vi "Driver Controller.vi"   [LabVIEW 2018]
uses:
  <vilib>/Rock Robotics/WPI/Joystick/WPI_JoystickDeviceEnum.ctl
  Driver Controller Global.vi
types:
  T1 = typedef "WPI_JoystickDeviceEnum.ctl" = enum16{"USB 0", "USB 1", "USB 2", "USB 3", "USB 4", "USB 5"}
  T2 = typedef "WPI_JoystickDevRef.ctl" = cluster{"Device":T1}
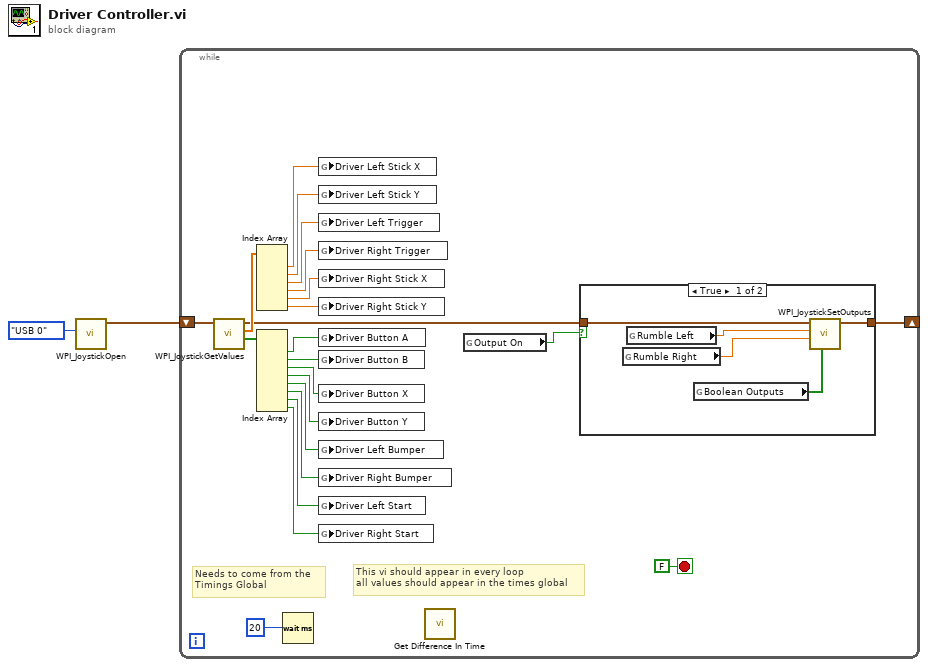
[diagram p0: block diagram]
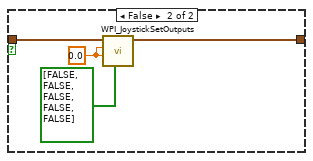
[diagram p2: hidden frame]
diagram:
  n1 = call <vilib>:"WPI_JoystickOpen.vi"("JoystickDevice"=WPI_JoystickDeviceEnum."USB 0") -> ("JoystickDevRef"=w1:T2)  [unwired: 10 in]
  n2 = while {
    shift-right: [w5] -> _
    shift-left: w1 -> [w24]
    stop <- FALSE stop-if-true
    # "This vi should appear in every loop\nall values should appear in the times global"
    # "Needs to come from the\nTimings Global"
    n3 = call <vilib>:"WPI_JoystickGetValues.vi"("JoystickDevRef"=w24) -> ("Buttons"=w16:bool[], "Axes"=w23:dbl[], "JoystickDevRef"=w4:T2)  [unwired: 6 in, 2 out]
    n4 = Index Array(array=w23) -> (element #1=w22:dbl, element #2=w21:dbl, element #3=w20:dbl, element #4=w19:dbl, element #5=w18:dbl, element #6=w17:dbl)  [unwired: 6 in]
    n5 = Index Array(array=w16) -> (element #1=w15:bool, element #2=w14:bool, element #3=w13:bool, element #4=w12:bool, element #5=w11:bool, element #6=w10:bool, element #7=w9:bool, element #8=w8:bool)  [unwired: 8 in]
    n6 = Wait (ms)(milliseconds to wait=20) -> ()  [unwired: 1 out]
    n7 = global write "Driver Controller Global.vi" "Driver Left Stick X"(w22) -> ()
    n8 = global write "Driver Controller Global.vi" "Driver Left Stick Y"(w21) -> ()
    n9 = global write "Driver Controller Global.vi" "Driver Left Trigger"(w20) -> ()
    n10 = global write "Driver Controller Global.vi" "Driver Right Trigger"(w19) -> ()
    n11 = global write "Driver Controller Global.vi" "Driver Right Stick X"(w18) -> ()
    n12 = global write "Driver Controller Global.vi" "Driver Right Stick Y"(w17) -> ()
    n13 = global write "Driver Controller Global.vi" "Driver Button A"(w15) -> ()
    n14 = global write "Driver Controller Global.vi" "Driver Button B"(w14) -> ()
    n15 = global write "Driver Controller Global.vi" "Driver Button X"(w13) -> ()
    n16 = global write "Driver Controller Global.vi" "Driver Button Y"(w12) -> ()
    n17 = global write "Driver Controller Global.vi" "Driver Left Bumper"(w11) -> ()
    n18 = global write "Driver Controller Global.vi" "Driver Right Bumper"(w10) -> ()
    n19 = global write "Driver Controller Global.vi" "Driver Left Start"(w9) -> ()
    n20 = global write "Driver Controller Global.vi" "Driver Right Start"(w8) -> ()
    n21 = call "Get Difference In Time.vi"() -> ()  [unwired: 10 in, 2 out]
    n22 = global read "Driver Controller Global.vi" "Output On"() -> (w3:bool)
    n23 = case shown="True" w3 {
      tunnel: [w29 w33] -> w5
      tunnel: w4 -> [w28 w32]
      frame True {
        n24 = global read "Driver Controller Global.vi" "Rumble Right"() -> (w26:dbl)
        n25 = global read "Driver Controller Global.vi" "Rumble Left"() -> (w27:dbl)
        n26 = global read "Driver Controller Global.vi" "Boolean Outputs"() -> (w25:bool[])
        n27 = call <vilib>:"WPI_JoystickSetOutputs.vi"("Outputs"=w25, "Right Rumble"=w26, "Left Rumble"=w27, "JoystickDevRef"=w28) -> ("JoystickDevRef"=w29:T2)  [unwired: 6 in, 1 out]
      }
      frame False {
        w31 = sgl 0.0 ("Left Rumble")
        n28 = call <vilib>:"WPI_JoystickSetOutputs.vi"("Outputs"=bool[] [FALSE, FALSE, FALSE, FALSE, FALSE], "Right Rumble"=w31, "Left Rumble"=w31, "JoystickDevRef"=w32) -> ("JoystickDevRef"=w33:T2)  [unwired: 6 in, 1 out]
      }
    }
  }
